vi "Update.vi"(8 "error in (no error)":errorcluster, 10 "Distance Travelled":dbl, 11 "MovementInstruction in":refnum<class "MovementInstruction.lvclass">) -> (0 "error out":errorcluster, 3 "MovementInstruction out":refnum<class "MovementInstruction.lvclass">)   [LabVIEW 2015, in "MovementInstruction.lvclass"]
uses:
  MovementInstruction.lvclass
  MovementInstruction.lvclass/MovementInstruction.ctl
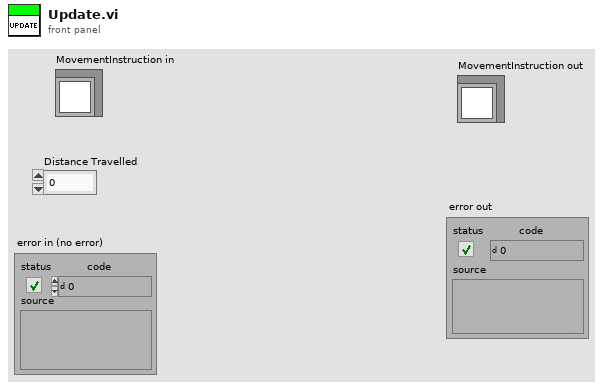
[diagram p1: front panel]
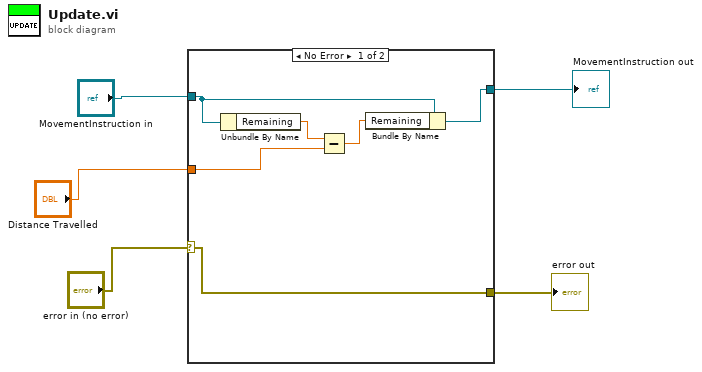
[diagram p0: block diagram]
diagram:
  n1 = case shown="No Error" "error in (no error)" {
    selector: "error in (no error)" -> [w6 w13]
    tunnel: [w6 w13] -> w4
    tunnel: "MovementInstruction in" -> [w11 w12]
    tunnel: [w10 w12] -> w2
    tunnel: "Distance Travelled" -> [w9 _]
    frame No Error {
      n2 = Unbundle By Name(w11) -> ("Remaining"=w8:dbl)
      n3 = Subtract(x=w8, y=w9) -> (x-y=w7:dbl)
      n4 = Bundle By Name(cluster=w11, "Remaining"=w7) -> (w10:refnum<class "MovementInstruction.lvclass">)
    }
    frame Error {
    }
  }
  "MovementInstruction out" <- w2
  "error out" <- w4
